vi "test.vi"() -> ()   [LabVIEW 2013]
uses:
  ReadingsCtrl.ctl
  <vilib>/express/express arith-compare/Formula/XNode/ExpressFormulaBlockNode.xnode
panel:
  out "Estimated I":dbl=10.0 caption="Est. Current [A]"
  in  "Increments":u16=10 caption="StepSize [A]"
  out "error out 17":errorcluster
  out "error out 16":errorcluster
  out "error out 15":errorcluster
  out "error in (no error) 3":errorcluster
  out "error in (no error) 2":errorcluster
  out "error out 14":errorcluster
  out "error out 13":errorcluster
  out "Message":string
  in  "dec":bool
  in  "inc":bool
  out "Mag ON OFF Status":bool
  in  "Remote Turn ONOFF":bool caption="Toggle to turn on"
  in  "HMI PWR":u16
  out "error out 12":errorcluster
  out "error out 11":errorcluster
  out "error out 10":errorcluster
  out "error out 9":errorcluster
  out "error out 8":errorcluster
  out "Readings":T1 {"COND" format="%.3f"}
  out "error out 7":errorcluster
  out "error out 6":errorcluster
  out "Interlock":bool
  out "Remote ON":bool
  out "TMP_IL":bool
  out "KLXON_IL":bool
  out "COND_IL":bool
  out "FLW_IL":bool
  out "error out 5":errorcluster
  out "error out 4":errorcluster
  out "error out 3":errorcluster
  out "error out 2":errorcluster
  out "error out":errorcluster
  in  "error in (no error)":errorcluster
  in  "stop":bool
  # "MagSpec Remote Monitoring and Control"
  # "Set Current [A]"
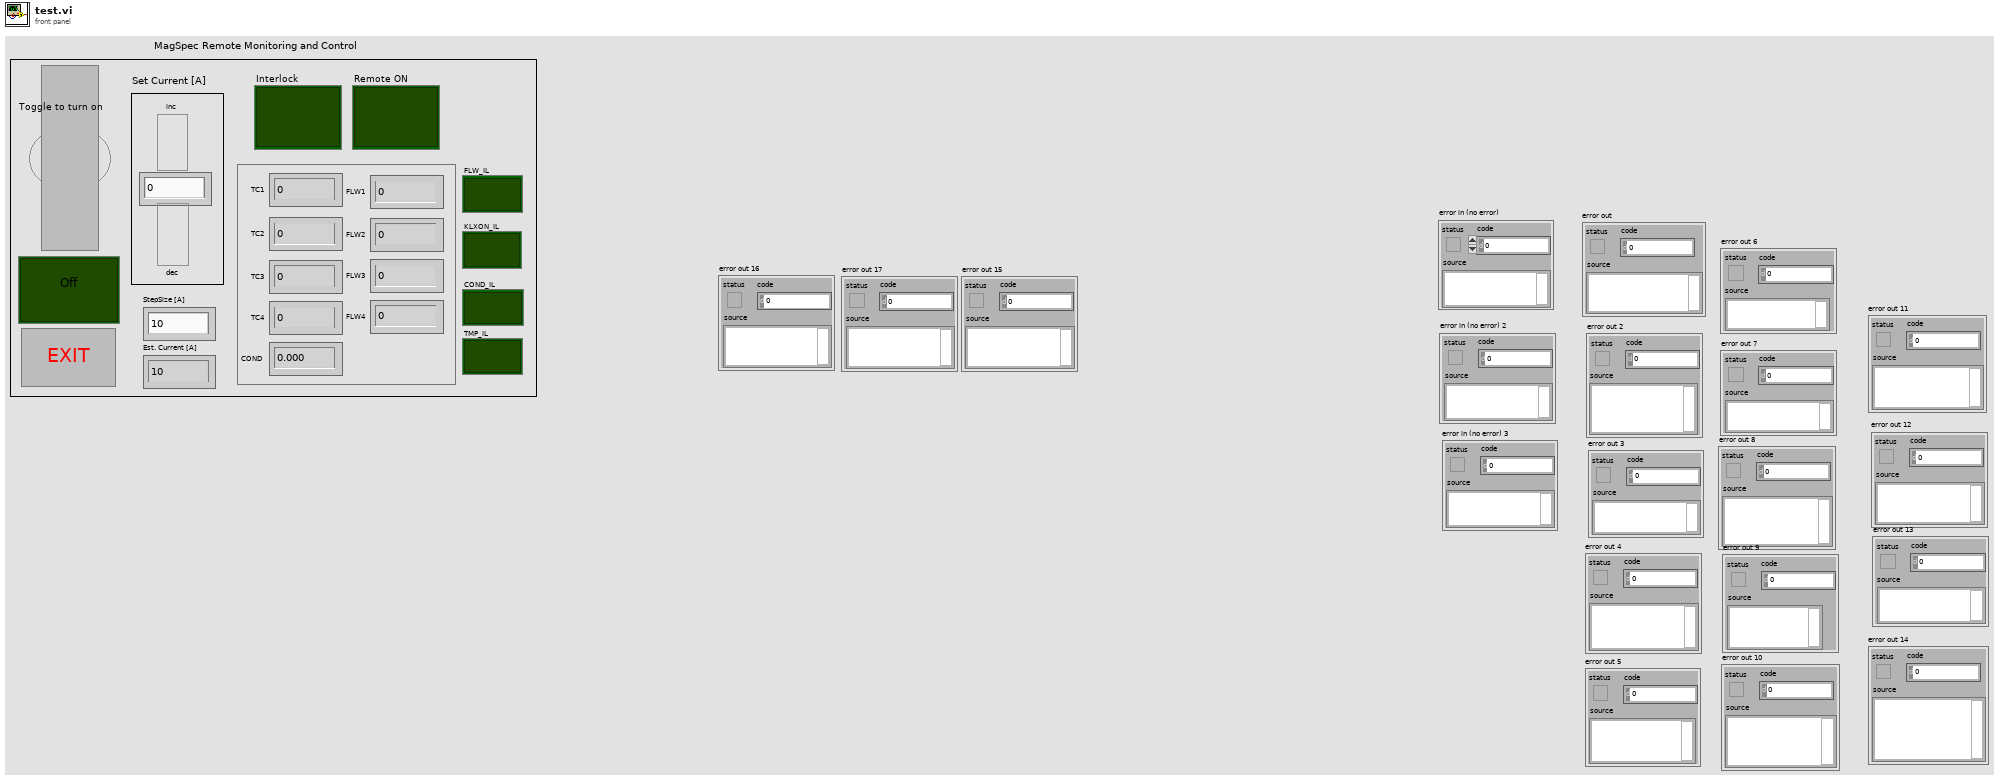
[diagram p1: front panel]
types:
  T1 = typedef "ReadingsCtrl.ctl" = cluster{"TC1":dbl, "TC2":dbl, "TC3":dbl, "TC4":dbl, "FLW1":dbl, "FLW2":dbl, "FLW3":dbl, "FLW4":dbl, "COND":dbl, "KLX1":bool, "KLX2":bool}
  T2 = cluster{"Enable Reset HMI":bool, "Power Val":u16}
  T3 = enum8{"Enabled", "Disabled", "Disabled and Grayed Out"}
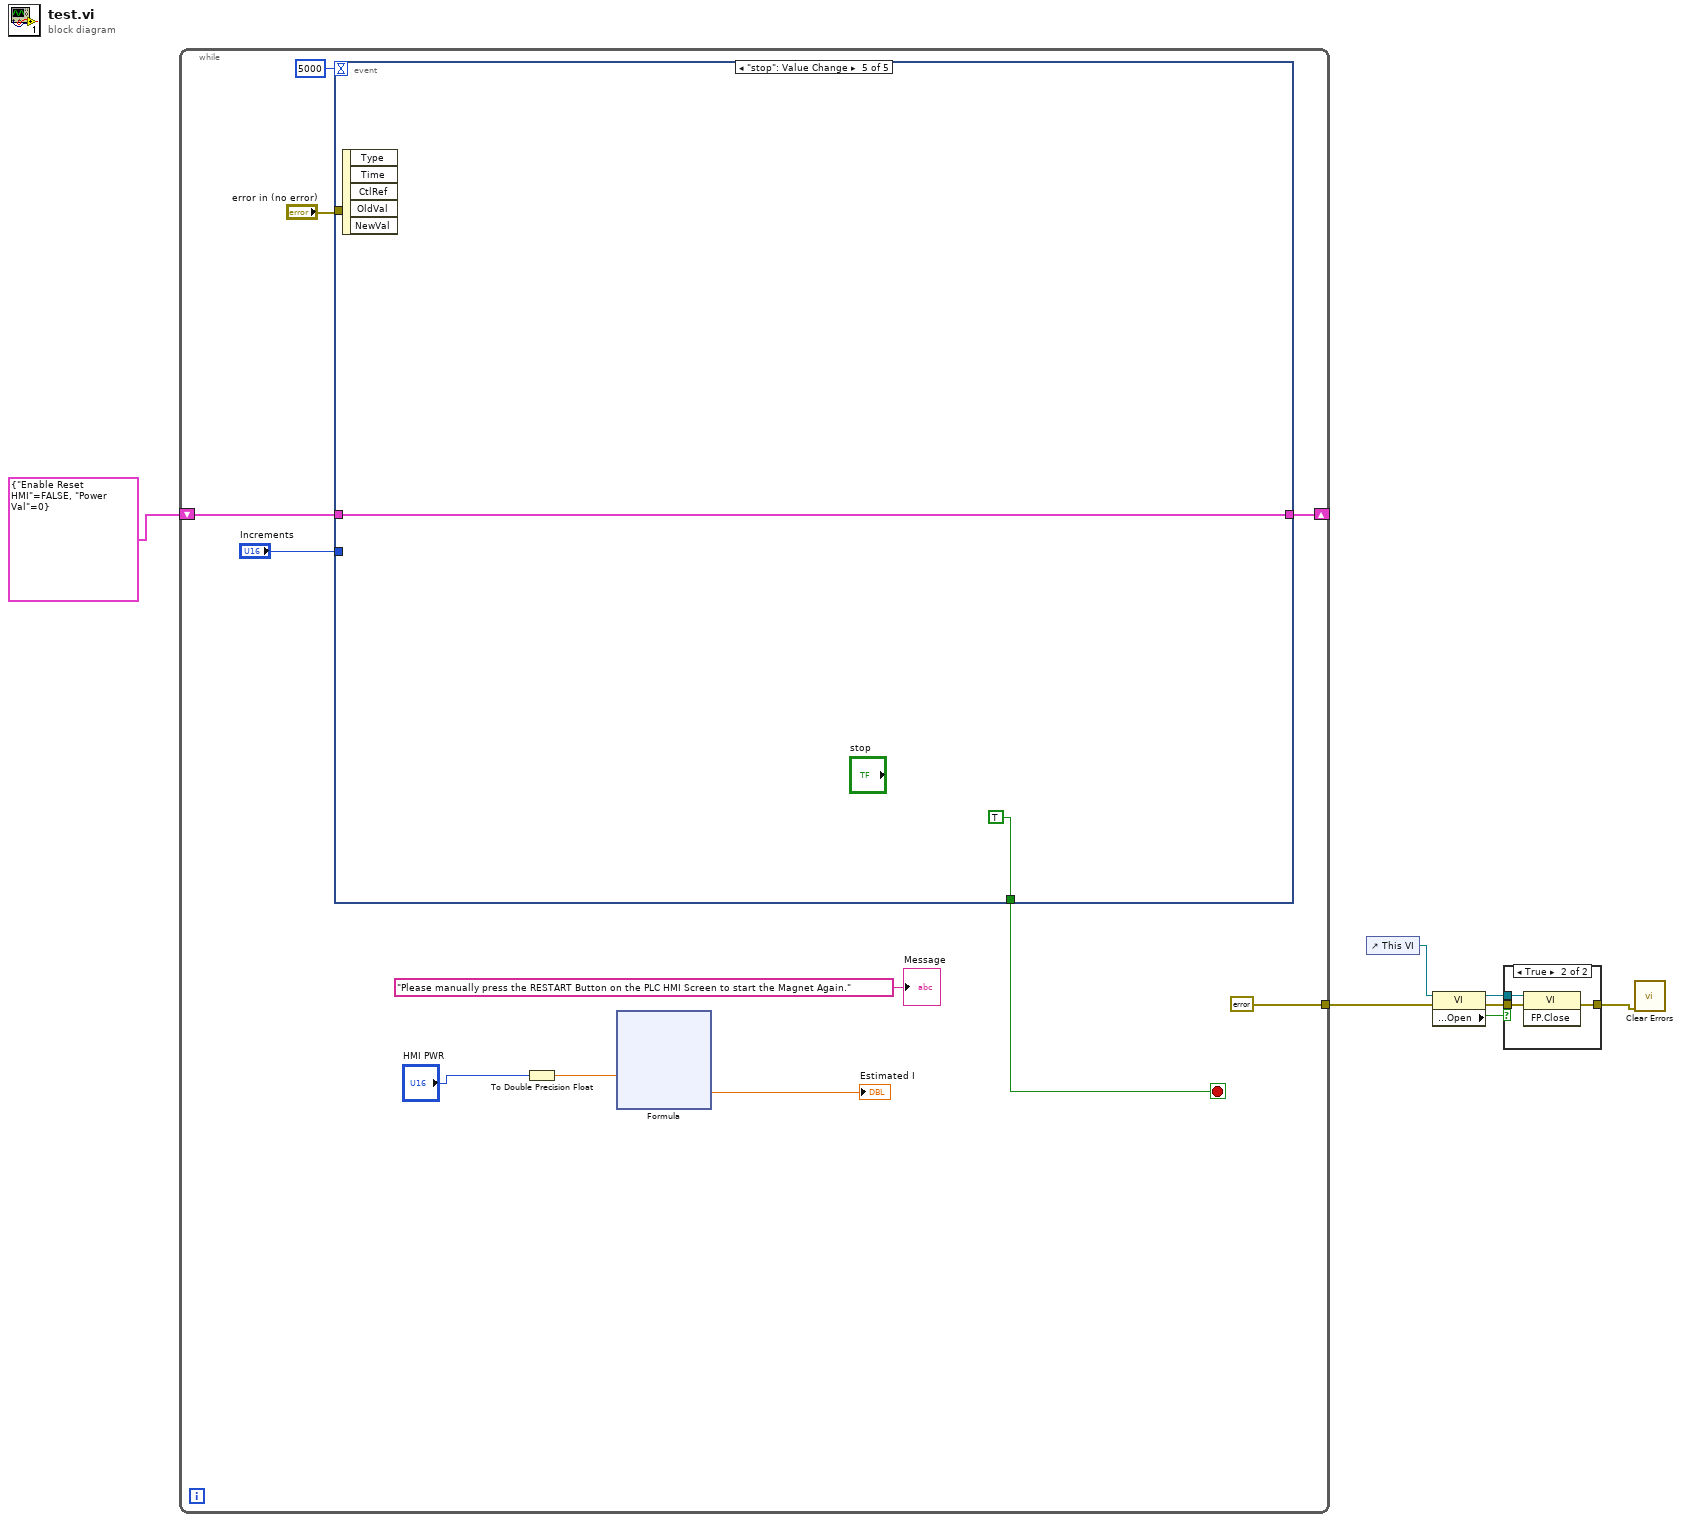
[diagram p0: block diagram]
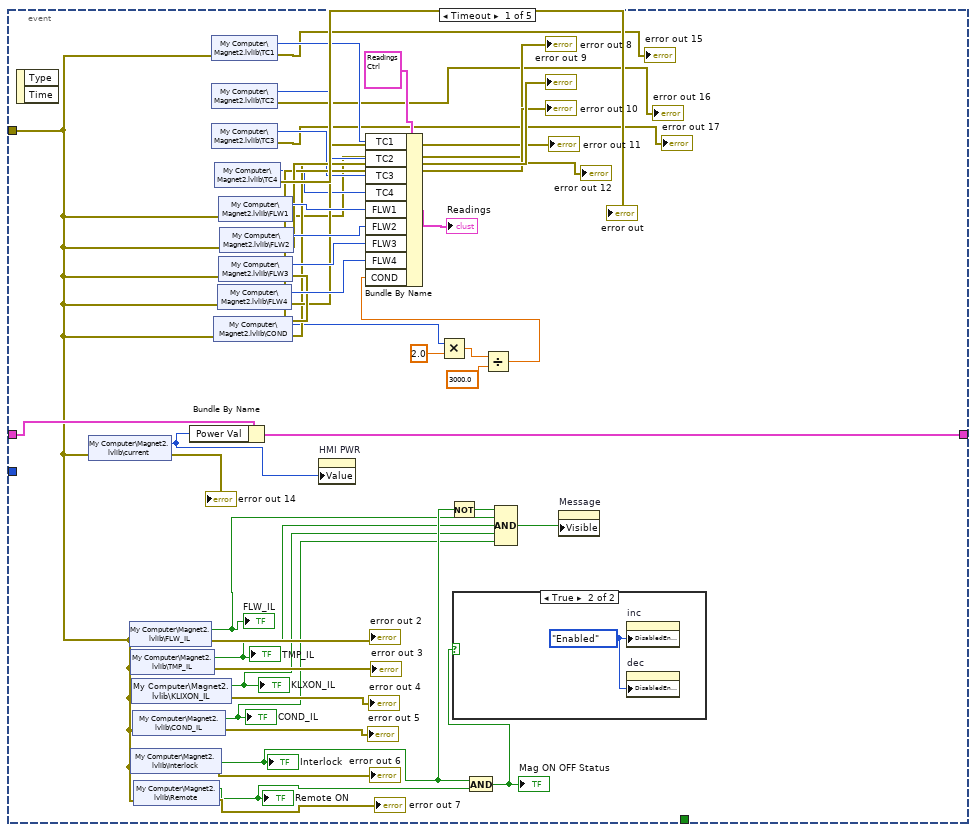
[diagram p3: hidden frame]
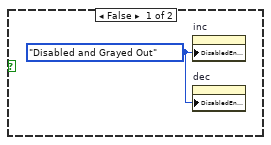
[diagram p4: hidden frame]
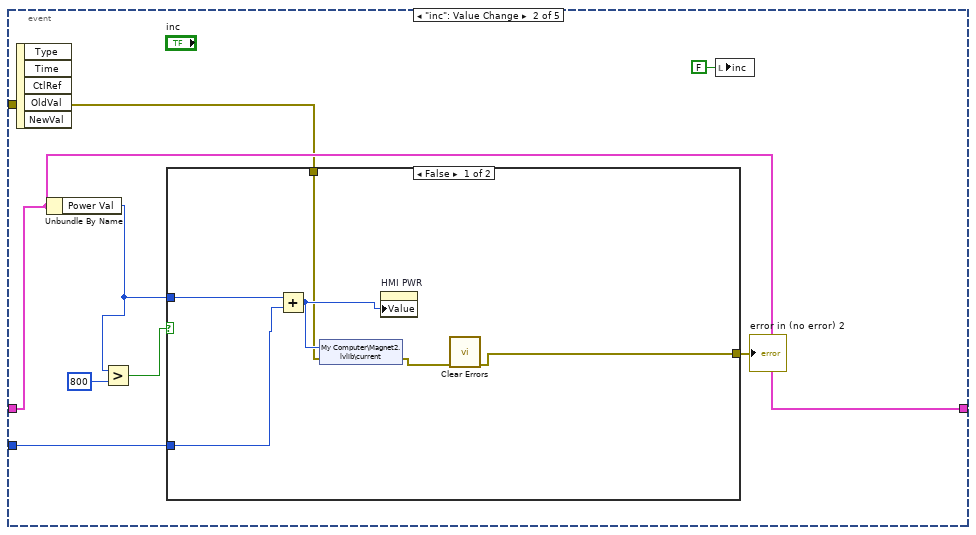
[diagram p5: hidden frame]
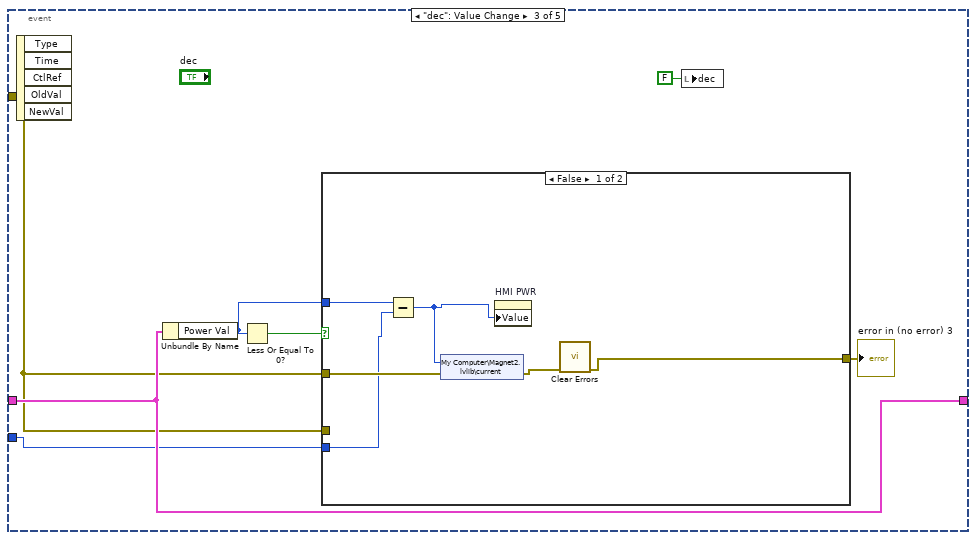
[diagram p7: hidden frame]
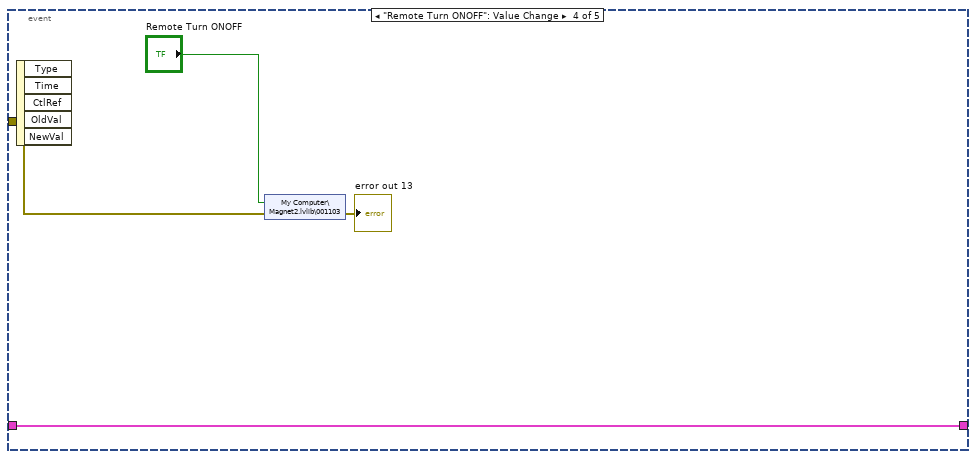
[diagram p9: hidden frame]
diagram:
  n1 = while {
    shift-right: [w13] -> _
    shift-left: T2 {"Enable Reset HMI"=FALSE, "Power Val"=0} -> [w14]
    tunnel: [errorcluster {"status"=FALSE, "code"=0, "source"=""} ("error in (no error)")] -> w1
    stop <- w17 stop-if-true
    n2 = event shown="[4] \"stop\": Value Change" {
      selector: _ -> [_ _ _ _ _]
      dyn-events: _ -> [_ _ _ _ _]
      timeout: 5000 -> [_ _ _ _ _]
      tunnel: "error in (no error)" -> [w37 w76 w91 w105 _]
      tunnel: [_ _ _ _ TRUE] -> w17
      tunnel: w14 -> [w39 w77 w92 w103 w106]
      tunnel: [w38 w77 w92 w103 w106] -> w13
      tunnel: "Increments" -> [_ w73 w88 _ _]
      event Timeout {
        n3 = event-data() -> ()  [unwired: 1 in, 2 out]
        n4 = shared-variable "My Computer\\Magnet2.lvlib\\current"(error in=w37) -> (w35:i32, error out=→"error out 14":errorcluster)
        n5 = shared-variable "My Computer\\Magnet2.lvlib\\FLW_IL"(error in=w37) -> (w45:bool, error out=→"error out 2":errorcluster)
        "FLW_IL" <- w45
        n6 = shared-variable "My Computer\\Magnet2.lvlib\\TMP_IL"(error in=w37) -> (w44:bool, error out=→"error out 3":errorcluster)
        "TMP_IL" <- w44
        n7 = shared-variable "My Computer\\Magnet2.lvlib\\Interlock"(error in=w37) -> (w46:bool, error out=→"error out 6":errorcluster)
        "Interlock" <- w46
        n8 = shared-variable "My Computer\\Magnet2.lvlib\\KLIXON_IL"(error in=w37) -> (w43:bool, error out=→"error out 4":errorcluster)
        "KLXON_IL" <- w43
        n9 = shared-variable "My Computer\\Magnet2.lvlib\\COND_IL"(error in=w37) -> (w42:bool, error out=→"error out 5":errorcluster)
        "COND_IL" <- w42
        n10 = shared-variable "My Computer\\Magnet2.lvlib\\Remote"(error in=w37) -> (w40:bool, error out=→"error out 7":errorcluster)
        "Remote ON" <- w40
        n11 = Bundle By Name(cluster=w39, "Power Val"=w35) -> (w38:T2)
        n12 = shared-variable "My Computer\\Magnet2.lvlib\\TC1"(error in=w37) -> (w54:u16, error out=→"error out 15":errorcluster)
        n13 = shared-variable "My Computer\\Magnet2.lvlib\\TC2"() -> (w53:u16, error out=→"error out 16":errorcluster)  [unwired: 1 in]
        n14 = shared-variable "My Computer\\Magnet2.lvlib\\TC3"() -> (w52:u16, error out=→"error out 17":errorcluster)  [unwired: 1 in]
        n15 = shared-variable "My Computer\\Magnet2.lvlib\\COND"(error in=w37) -> (w34:u16, error out=→"error out 12":errorcluster)
        n16 = shared-variable "My Computer\\Magnet2.lvlib\\TC4"() -> (w51:u16, error out=→"error out":errorcluster)  [unwired: 1 in]
        n17 = shared-variable "My Computer\\Magnet2.lvlib\\FLW4"(error in=w37) -> (w58:u16, error out=→"error out 11":errorcluster)
        n18 = shared-variable "My Computer\\Magnet2.lvlib\\FLW1"(error in=w37) -> (w61:u16, error out=→"error out 8":errorcluster)
        n19 = shared-variable "My Computer\\Magnet2.lvlib\\FLW3"(error in=w37) -> (w59:u16, error out=→"error out 10":errorcluster)
        n20 = shared-variable "My Computer\\Magnet2.lvlib\\FLW2"(error in=w37) -> (w60:u16, error out=→"error out 9":errorcluster)
        n21 = property on="HMI PWR" class="DigNum (strict)"("Value"=w35) -> ()  [unwired: 2 in, 2 out]
        n22 = Multiply(x=w34, y=2.0) -> (x*y=w32:dbl)
        n23 = Not(x=w46) -> (.not. x?=w47:bool)
        n24 = And(x=w46, y=w40) -> (x .and. y?=w48:bool)
        "Mag ON OFF Status" <- w48
        n25 = case shown="True" w48 {
          frame False {
            w71 = T3."Disabled and Grayed Out" ("Disabled")
            n26 = property on="inc" class="Bool (strict)"("DisabledEnum"=w71) -> ()  [unwired: 2 in, 2 out]
            n27 = property on="dec" class="Bool (strict)"("DisabledEnum"=w71) -> ()  [unwired: 2 in, 2 out]
          }
          frame True {
            w72 = T3."Enabled" ("Disabled")
            n28 = property on="inc" class="Bool (strict)"("DisabledEnum"=w72) -> ()  [unwired: 2 in, 2 out]
            n29 = property on="dec" class="Bool (strict)"("DisabledEnum"=w72) -> ()  [unwired: 2 in, 2 out]
          }
        }
        n30 = Divide(x=w32, y=3000.0) -> (x/y=w30:dbl)
        n31 = Bundle By Name(cluster=T1 {"TC1"=0.0, "TC2"=0.0, "TC3"=0.0, "TC4"=0.0, "FLW1"=0.0, "FLW2"=0.0, "FLW3"=0.0, "FLW4"=0.0, "COND"=0.0, "KLX1"=FALSE, "KLX2"=FALSE} ("Readings"), "TC1"=w54, "TC2"=w53, "TC3"=w52, "TC4"=w51, "FLW1"=w61, "FLW2"=w60, "FLW3"=w59, "FLW4"=w58, "COND"=w30) -> (→"Readings":T1)
        n32 = Compound Arithmetic op=AND(w47, w45, w44, w43, w42) -> (w41:bool)
        n33 = property on="Message" class="Str"("Visible"=w41) -> ()  [unwired: 2 in, 2 out]
      }
      event "inc": Value Change {
        n34 = event-data() -> ()  [unwired: 1 in, 5 out]
        n35 = Unbundle By Name(w77) -> ("Power Val"=w80:u16)
        n36 = Greater?(x=w80, y=u16 800) -> (0:w79:bool)
        n37 = case shown="False" w79 {
          tunnel: w80 -> [w86 _]
          tunnel: [w85 w87] -> w75
          tunnel: w76 -> [w83 w87]
          tunnel: w73 -> [w81 _]
          frame False {
            n38 = Add(x=w86, y=w81) -> (x+y=w84:u16)
            n39 = shared-variable "My Computer\\Magnet2.lvlib\\current"(w84, error in=w83) -> (error out=w82:errorcluster)
            n40 = property on="HMI PWR" class="DigNum (strict)"("Value"=w84) -> ()  [unwired: 2 in, 2 out]
            n41 = call <vilib>:"Clear Errors.vi"("error in (no error)"=w82) -> ("error out"=w85:errorcluster)  [unwired: 6 in]
          }
          frame True {
          }
        }
        "error in (no error) 2" <- w75
        n42 = local write "inc"(FALSE ("inc")) -> ()
      }
      event "dec": Value Change {
        n43 = event-data() -> ()  [unwired: 1 in, 5 out]
        n44 = Unbundle By Name(w92) -> ("Power Val"=w94:u16)
        n45 = Less Or Equal To 0?(x=w94) -> (x <= 0?=w93:bool)
        n46 = case shown="False" w93 {
          tunnel: w94 -> [w100 _]
          tunnel: [w99 w101] -> w90
          tunnel: w91 -> [_ w101]
          tunnel: w91 -> [w96 _]
          tunnel: w88 -> [w95 _]
          frame False {
            n47 = Subtract(x=w100, y=w95) -> (x-y=w98:u16)
            n48 = shared-variable "My Computer\\Magnet2.lvlib\\current"(w98, error in=w96) -> (error out=w97:errorcluster)
            n49 = property on="HMI PWR" class="DigNum (strict)"("Value"=w98) -> ()  [unwired: 2 in, 2 out]
            n50 = call <vilib>:"Clear Errors.vi"("error in (no error)"=w97) -> ("error out"=w99:errorcluster)  [unwired: 6 in]
          }
          frame True {
            # "Do not set value below zero"
          }
        }
        "error in (no error) 3" <- w90
        n51 = local write "dec"(FALSE ("dec")) -> ()
      }
      event "Remote Turn ONOFF": Value Change {
        n52 = event-data() -> ()  [unwired: 1 in, 5 out]
        n53 = shared-variable "My Computer\\Magnet2.lvlib\\001103"("Remote Turn ONOFF", error in=w105) -> (error out=→"error out 13":errorcluster)
      }
      event "stop": Value Change {
        n54 = event-data() -> ()  [unwired: 1 in, 5 out]
      }
    }
    n55 = To Double Precision Float(number="HMI PWR") -> (double precision float=w9:dbl)
    n56 = xnode "Formula"("X1"=w9) -> ("Result"=→"Estimated I":dbl)  [unwired: 1 in, 1 out]
    "Message" <- "Please manually press the RESTART Button on the PLC HMI Screen to start the Magnet Again." ("String")
  }
  n57 = control-ref of="This VI"() -> (w3:refnum<vi>)
  n58 = property class="VI"(reference=w3, error in=w1) -> (reference out=w5:refnum<vi>, error out=w6:errorcluster, "Front Panel.Open"=w4:bool)
  n59 = case shown="True" w4 {
    tunnel: [w108 w111] -> w2
    tunnel: w6 -> [w108 w110]
    tunnel: w5 -> [_ w109]
    frame False {
    }
    frame True {
      n60 = invoke class="VI" method="FP.Close"(reference=w109, error in=w110) -> (error out=w111:errorcluster)  [unwired: 1 in, 2 out]
    }
  }
  n61 = call <vilib>:"Clear Errors.vi"("error in (no error)"=w2) -> ()  [unwired: 6 in, 1 out]
